vi "AutoNamerConfigNew.vi"(2 "Custom Folder":string, 3 "User Data Folder":T1) -> (0 "Data file":string, 1 "Path":path)   [LabVIEW 2014]
uses:
  Users/mbcsslp2/Control 1.ctl
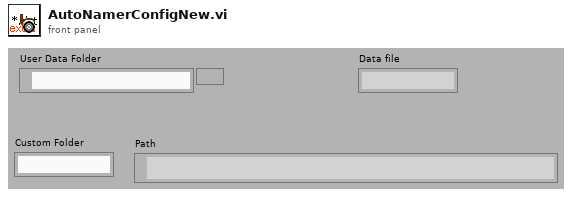
[diagram p1: front panel]
types:
  T1 = typedef "Control 1.ctl" = path
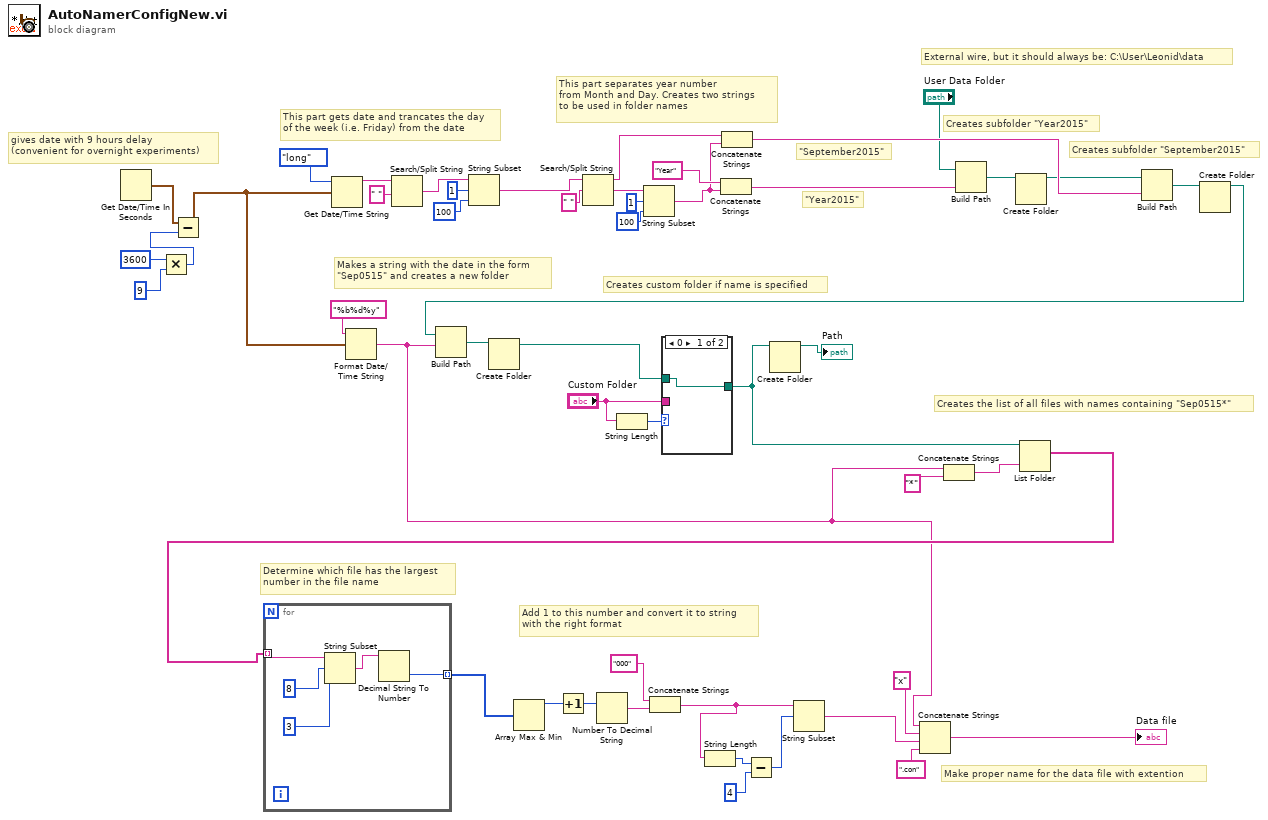
[diagram p0: block diagram]
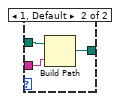
[diagram p2: hidden frame]
diagram:
  # "Add 1 to this number and convert it to string\nwith the right format"
  # "Determine which file has the largest \nnumber in the file name"
  # "External wire, but it should always be: C:\\User\\Leonid\\data"
  # "Make proper name for the data file with extention"
  # "Creates the list of all files with names containing \"Sep0515*\""
  # "Creates custom folder if name is specified"
  # "Makes a string with the date in the form \n\"Sep0515\" and creates a new folder"
  # "Creates subfolder \"September2015\""
  # "Creates subfolder \"Year2015\""
  # "\"September2015\""
  # "\"Year2015\""
  # "This part separates year number \nfrom Month and Day. Creates two strings\nto be used in folder names"
  # "This part gets date and trancates the day \nof the week (i.e. Friday) from the date"
  # "gives date with 9 hours delay\n(convenient for overnight experiments)"
  n1 = Get Date/Time In Seconds() -> (seconds since 1Jan1904=w22:timestamp)
  n2 = Multiply(x=3600, y=9) -> (x*y=w19:i32)
  n3 = Subtract(x=w22, y=w19) -> (x-y=w16:timestamp)
  n4 = Get Date/Time String(date format (0)=enum16{"short", "long", "abbreviated"}."long", seconds (now)=w16) -> (date string=w46:string)  [unwired: 1 in, 1 out]
  n5 = Format Date/Time String(time format string (%c)="%b%d%y", seconds (now)=w16) -> (date/time string=w2:string)  [unwired: 1 in]
  n6 = Search/Split String(string=w46, search string/char (-)=" ") -> (match + rest of string=w44:string)  [unwired: 1 in, 2 out]
  n7 = String Subset(string=w44, offset (0)=1, length (rest)=100 ("length (rest)")) -> (substring=w37:string)
  n8 = Search/Split String(string=w37, search string/char (-)=" ") -> (substring before match=w33:string, match + rest of string=w38:string)  [unwired: 1 in, 1 out]
  n9 = String Length(string="Custom Folder") -> (length=w18:i32)
  n10 = String Subset(string=w38, offset (0)=1, length (rest)=100 ("length (rest)")) -> (substring=w34:string)
  n11 = Concatenate Strings("Year" ("Substring"), w34) -> (w35:string)
  n12 = Concatenate Strings(w33, w34) -> (w32:string)
  n13 = Concatenate Strings(w2, "*") -> (w49:string)
  n14 = Build Path(base path="User Data Folder", name or relative path=w35) -> (appended path=w31:path)
  n15 = Create Folder(path (use dialog)=w31) -> (created path=w30:path)  [unwired: 2 in, 2 out]
  n16 = Build Path(base path=w30, name or relative path=w32) -> (appended path=w29:path)
  n17 = Create Folder(path (use dialog)=w29) -> (created path=w28:path)  [unwired: 2 in, 2 out]
  n18 = Build Path(base path=w28, name or relative path=w2) -> (appended path=w23:path)
  n19 = Create Folder(path (use dialog)=w23) -> (created path=w24:path)  [unwired: 2 in, 2 out]
  n20 = case shown="0" w18 {
    tunnel: [w51 w54] -> w25
    tunnel: w24 -> [w51 w53]
    tunnel: "Custom Folder" -> [_ w52]
    frame 0 {
    }
    frame 1, Default {
      n21 = Build Path(base path=w53, name or relative path=w52) -> (appended path=w54:path)
    }
  }
  n22 = Create Folder(path (use dialog)=w25) -> (created path=→"Path":path)  [unwired: 2 in, 2 out]
  n23 = List Folder(path=w25, pattern=w49) -> (filenames=w15:string[])  [unwired: 2 in, 3 out]
  n24 = for {
    tunnel: w15 -> [w59] mode=indexing
    tunnel: [w55] -> w14 mode=indexing
    n25 = String Subset(string=w59, offset (0)=8, length (rest)=3) -> (substring=w56:string)
    n26 = Decimal String To Number(string=w56) -> (number=w55:i32)  [unwired: 2 in, 1 out]
  }
  n27 = Array Max & Min(array=w14) -> (max value=w13:i32)  [unwired: 3 out]
  n28 = Increment(x=w13) -> (x+1=w12:i32)
  n29 = Number To Decimal String(number=w12) -> (decimal integer string=w11:string)  [unwired: 1 in]
  n30 = Concatenate Strings("000", w11) -> (w6:string)
  n31 = String Length(string=w6) -> (length=w9:i32)
  n32 = Subtract(x=w9, y=4) -> (x-y=w7:i32)
  n33 = String Subset(string=w6, offset (0)=w7) -> (substring=w3:string)  [unwired: 1 in]
  n34 = Concatenate Strings(w2, "x", w3, ".con" ("Substring")) -> (→"Data file":string)
